vi "Write Config File.vi"(8 "error in (no error)":errorcluster, 10 "ConfigFile":path, 11 "Options":T1) -> (0 "error out":errorcluster)   [LabVIEW 2011]
uses:
  Controls/Options DVR.ctl
  Controls/Options.ctl
  <vilib>/Utility/config.llb/Write Key (Path).vi
  <vilib>/Utility/config.llb/Write Key (Boolean).vi
  <vilib>/Utility/config.llb/NI_LVConfig.lvlib
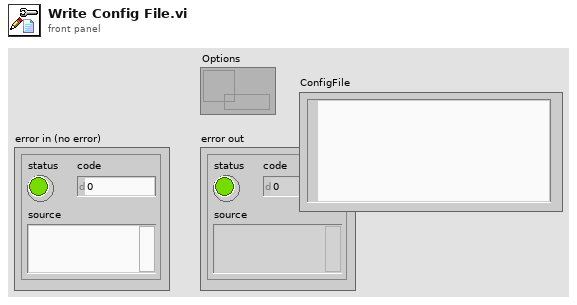
[diagram p1: front panel]
types:
  T1 = typedef "Options DVR.ctl" = refnum<data-value>
  T2 = typedef "Options.ctl" = cluster{"Logging?":bool, "TimeStamp?":bool, "LogInCSVDir?":bool, "LogDir":path}
  T3 = typedef "NI_LVConfig.lvlib/Config Data RefNum.ctl" = refnum<k1>
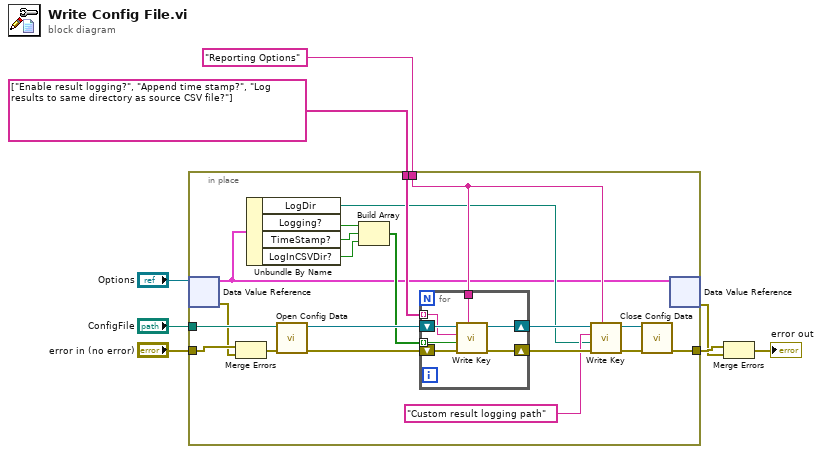
[diagram p0: block diagram]
diagram:
  n1 = in-place {
    in-place-border: string[] ["Enable result logging?", "Append time stamp?", "Log results to same directory as source CSV file?"] -> [w26]
    in-place-border: "Reporting Options" ("section") -> [w20]
    in-place-border: "error in (no error)" -> [w16]
    in-place-border: "ConfigFile" -> [w19]
    in-place-border: [w18] -> w3
    n2 = in-place-dvr #1("Options") -> (w9:T2, w15:errorcluster)
    n3 = Merge Errors(w16, w15) -> (w17:errorcluster)
    n4 = Unbundle By Name(w9) -> ("LogDir"=w14:path, "Logging?"=w11:bool, "TimeStamp?"=w12:bool, "LogInCSVDir?"=w13:bool)
    n5 = call <vilib>:"Open Config Data.vi"("error in (no error)"=w17, "configuration file path"=w19) -> ("error out"=w28:errorcluster, "refnum"=w27:T3)  [unwired: 7 in, 1 out]
    n6 = Build Array(w11, w12, w13) -> (w10:bool[])
    n7 = for {
      shift-right: [w33] -> w25
      shift-left: w28 -> [w35]
      shift-right: [w32] -> w24
      shift-left: w27 -> [w34]
      tunnel: w20 -> [w31]
      tunnel: w26 -> [w30] mode=indexing
      tunnel: w10 -> [w29] mode=indexing
      n8 = call-poly <vilib>:"Write Key.vi"("section"=w31, "error in (no error)"=w35, "value"=w29, "key"=w30, "refnum"=w34) -> ("error out"=w33:errorcluster, "refnum out"=w32:T3)  [unwired: 4 in, 1 out]
    }
    n9 = call-poly <vilib>:"Write Key.vi"("section"=w20, "error in (no error)"=w25, "value"=w14, "key"="Custom result logging path" ("section"), "refnum"=w24) -> ("error out"=w22:errorcluster, "refnum out"=w23:T3)  [unwired: 4 in, 1 out]
    n10 = call <vilib>:"Close Config Data.vi"("error in (no error)"=w22, "refnum"=w23) -> ("error out"=w18:errorcluster)  [unwired: 8 in, 1 out]
    n11 = in-place-dvr #1(w9) -> (w2:errorcluster)  [unwired: 1 out]
  }
  n12 = Merge Errors(w3, w2) -> (→"error out":errorcluster)
